vi "shutter-control.vi"() -> ()   [LabVIEW 2014]
uses:
  Shutter SubVis/ctts/laser shutters.ctl
  Shutter SubVis/ctts/user event shutter global.ctl
  Shutter SubVis/Global Shutter Variables - SubVI.vi
panel:
  out "Status":bool
  in  "Camera Shutter":bool
  in  "stop":bool
  in  "Laser Shutter":T1
  out "Current Wheel Position":string
  in  "Wheel Speed":u8=1 min=1 max=7 step=1
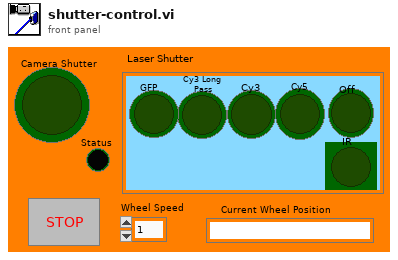
[diagram p1: front panel]
types:
  T1 = typedef "laser shutters.ctl" = enum32{"No Selection", "GFP", "Cy3 Long \nPass", "Cy3", "Cy5", "Off", "IR"}
  T2 = typedef "user event shutter global.ctl" = cluster{"Camera Shutter":bool, "Laser Shutter":enum32{"No Selection", "GFP", "Cy3 Long \nPass", "Cy3", "Cy5", "Off", "IR"}}
  T3 = enum32{"No Selection", "GFP", "Cy3 Long \nPass", "Cy3", "Cy5", "Off", "IR"}
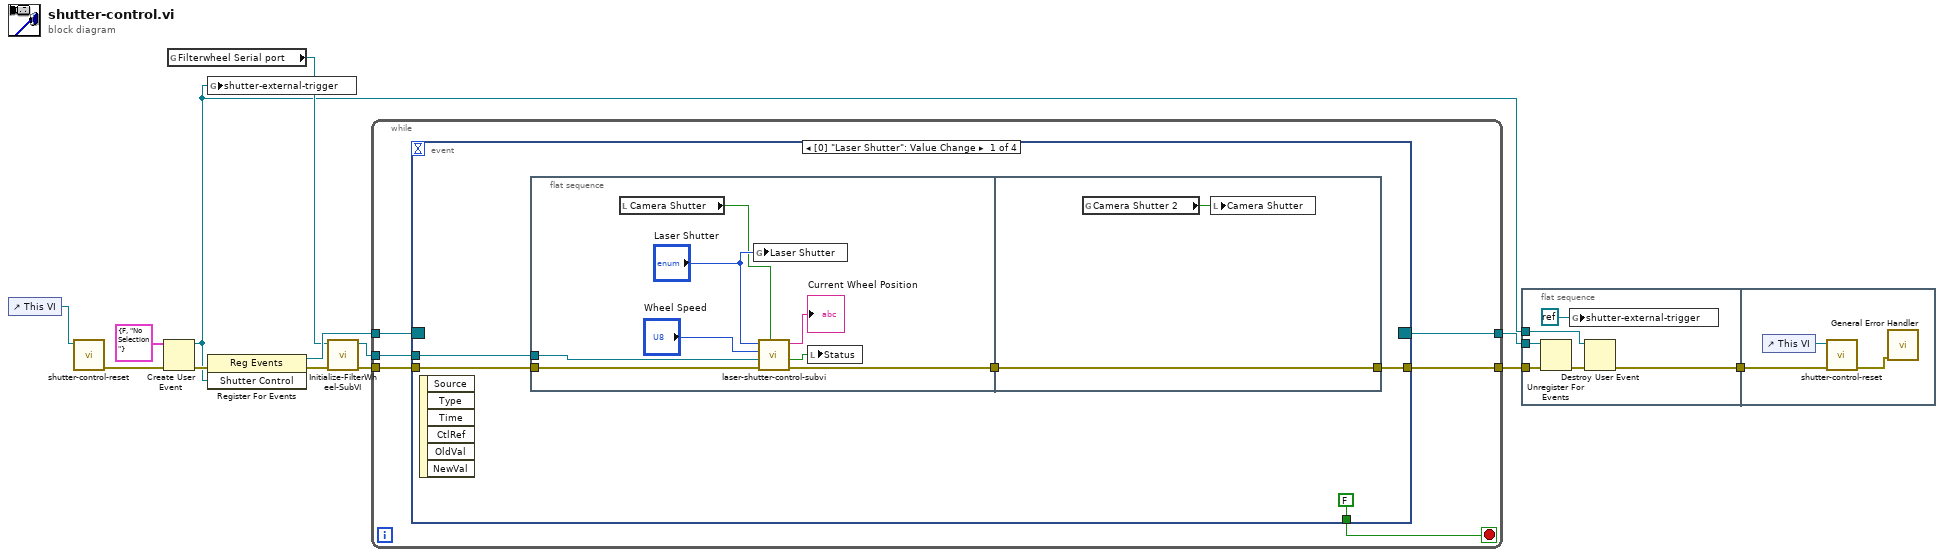
[diagram p0: block diagram]
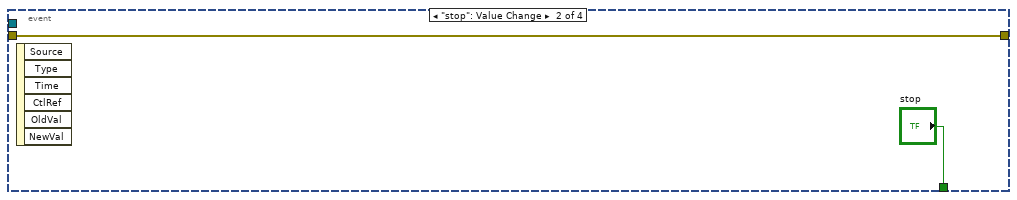
[diagram p2: hidden frame]
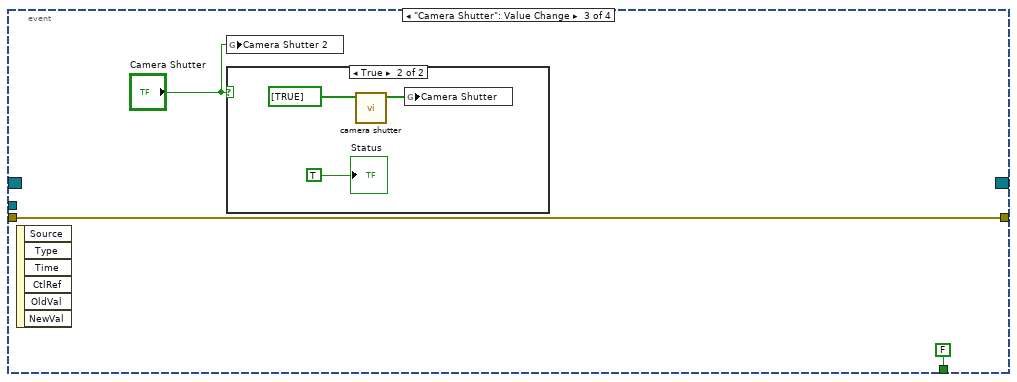
[diagram p3: hidden frame]
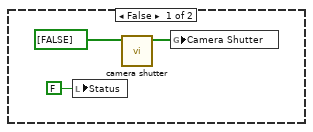
[diagram p4: hidden frame]
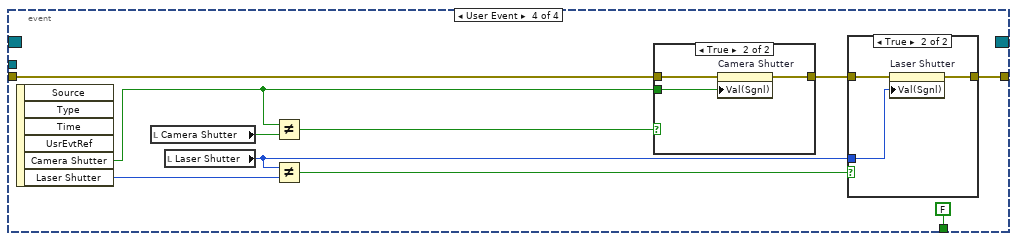
[diagram p5: hidden frame]
diagram:
  n1 = control-ref of="This VI"() -> (w4:refnum<vi>)
  n2 = call "shutter-control-reset.vi"("reference"=w4) -> ("error out"=w5:errorcluster)  [unwired: 10 in]
  n3 = Create User Event(user event datatype=T2 {"Camera Shutter"=FALSE, "Laser Shutter"=enum."No Selection"} ("Shutter Control"), error in=w5) -> (user event=w1:refnum<user-event>, error out=w12:errorcluster)
  n4 = global read "Global Shutter Variables - SubVI.vi" "Filterwheel Serial port"() -> (w2:refnum<visa-resource-name>)
  n5 = global write "Global Shutter Variables - SubVI.vi" "shutter-external-trigger"(w1) -> ()
  n6 = register-events(error in=w12, w1) -> (reference out=w11:refnum<event-registration>, error out=w8:errorcluster)  [unwired: 1 in]
  n7 = call "Initialize-FilterWheel-SubVI.vi"("Serial port"=w2, "error in"=w8) -> ("VISA resource name out"=w6:refnum<visa-resource-name>, "error out"=w7:errorcluster)  [unwired: 7 in]
  n8 = while {
    tunnel: [w16] -> w13
    tunnel: w7 -> [w17]
    tunnel: w11 -> [w19]
    tunnel: [w15] -> w10
    tunnel: w6 -> [w18]
    stop <- w14 stop-if-true
    n9 = event shown="[0] \"Laser Shutter\": Value Change" {
      selector: w19 -> [_ _ _ _]
      dyn-events: [_ _ _ _] -> w15
      timeout: _ -> [_ _ _ _]
      tunnel: w17 -> [w24 w35 w39 w50]
      tunnel: [w23 w35 w39 w47] -> w16
      tunnel: w18 -> [w22 _ _ _]
      tunnel: [FALSE ("stop") "stop" FALSE ("stop") FALSE ("stop")] -> w14
      event Value Change {
        n10 = event-data() -> ()  [unwired: 1 in, 6 out]
        n11 = flat-sequence {
          tunnel: w24 -> [w32]
          tunnel: w22 -> [w29]
          tunnel: [w31] -> w21
          tunnel: [w34] -> w23
          tunnel: w21 -> [w34]
          frame #0 {
            n12 = local read "Camera Shutter"() -> (w26:bool)
            n13 = global write "Global Shutter Variables - SubVI.vi" "Laser Shutter"("Laser Shutter") -> ()
            n14 = call "laser-shutter-control-subvi.vi"("Camera Shutter"=w26, "error in"=w32, "VISA resource name out"=w29, "Wheel Speed"="Wheel Speed", "Laser Shutter"="Laser Shutter") -> ("error out"=w31:errorcluster, "Status"=w25:bool, "Current Filterwheel"=→"Current Wheel Position":string)  [unwired: 4 in]
            n15 = local write "Status"(w25) -> ()
          }
          frame #1 {
            n16 = global read "Global Shutter Variables - SubVI.vi" "Camera Shutter 2"() -> (w33:bool)
            n17 = local write "Camera Shutter"(w33) -> ()
          }
        }
      }
      event "stop": Value Change {
        n18 = event-data() -> ()  [unwired: 1 in, 6 out]
      }
      event "Camera Shutter": Value Change {
        n19 = event-data() -> ()  [unwired: 1 in, 6 out]
        n20 = global write "Global Shutter Variables - SubVI.vi" "Camera Shutter 2"("Camera Shutter") -> ()
        n21 = case shown="True" "Camera Shutter" {
          frame False {
            n22 = local write "Status"(FALSE) -> ()
            n23 = call "camera shutter.vi"("Camera Input Switch"=bool[] [FALSE]) -> ("Camera Output Switch"=w42:bool[])  [unwired: 10 in]
            n24 = global write "Global Shutter Variables - SubVI.vi" "Camera Shutter"(w42) -> ()
          }
          frame True {
            n25 = call "camera shutter.vi"("Camera Input Switch"=bool[] [TRUE]) -> ("Camera Output Switch"=w44:bool[])  [unwired: 10 in]
            n26 = global write "Global Shutter Variables - SubVI.vi" "Camera Shutter"(w44) -> ()
            "Status" <- TRUE
          }
        }
      }
      event User Event {
        n27 = event-data() -> ("Camera Shutter"=w49:bool, "Laser Shutter"=w51:T3)  [unwired: 1 in, 4 out]
        n28 = local read "Camera Shutter"() -> (w54:bool)
        n29 = local read "Laser Shutter"() -> (w48:T1)
        n30 = Not Equal?(x=w49, y=w54) -> (x != y?=w55:bool)
        n31 = Not Equal?(x=w48, y=w51) -> (x != y?=w53:bool)
        n32 = case shown="True" w55 {
          tunnel: w49 -> [_ w63]
          tunnel: w50 -> [w60 w62]
          tunnel: [w60 w61] -> w52
          frame False {
          }
          frame True {
            n33 = property on="Camera Shutter" class="Bool (strict)"(error in=w62, "Val(Sgnl)"=w63) -> (error out=w61:errorcluster)  [unwired: 1 in, 1 out]
          }
        }
        n34 = case shown="True" w53 {
          tunnel: w52 -> [w56 w58]
          tunnel: w48 -> [_ w59]
          tunnel: [w56 w57] -> w47
          frame False {
          }
          frame True {
            n35 = property on="Laser Shutter" class="RadioBtnsControl (strict)"(error in=w58, "Val(Sgnl)"=w59) -> (error out=w57:errorcluster)  [unwired: 1 in, 1 out]
          }
        }
      }
    }
  }
  n36 = flat-sequence {
    tunnel: w13 -> [w68]
    tunnel: [w67] -> w3
    tunnel: w1 -> [w66]
    tunnel: w10 -> [w65]
    tunnel: w3 -> [w72]
    frame #0 {
      n37 = Unregister For Events(event registration refnum=w65, error in=w68) -> (error out=w69:errorcluster)
      n38 = global write "Global Shutter Variables - SubVI.vi" "shutter-external-trigger"(refnum<k0> refnum) -> ()
      n39 = Destroy User Event(user event=w66, error in=w69) -> (error out=w67:errorcluster)
    }
    frame #1 {
      n40 = control-ref of="This VI"() -> (w71:refnum<vi>)
      n41 = call "shutter-control-reset.vi"("error in"=w72, "reference"=w71) -> ("error out"=w70:errorcluster)  [unwired: 9 in]
      n42 = call <vilib>:"General Error Handler.vi"("error in (no error)"=w70) -> ()  [unwired: 10 in, 5 out]
    }
  }
